vi "Power vs. MW contrast scan.vi"() -> ()   [LabVIEW 2011]
uses:
  Colton LabView code/Instruments/Laser power controller/BEOC LPC/BEOC LPC.lvlib
panel:
  out "XY Graph":cluster{"Y":dbl[], "Y":dbl[]}[](graph)
  in  "Time(s)":dbl
  in  "Power Step":dbl
  in  "Power Max":dbl
  in  "Power Min":dbl
  in  "rate":dbl=100.0 format="%0.2f"
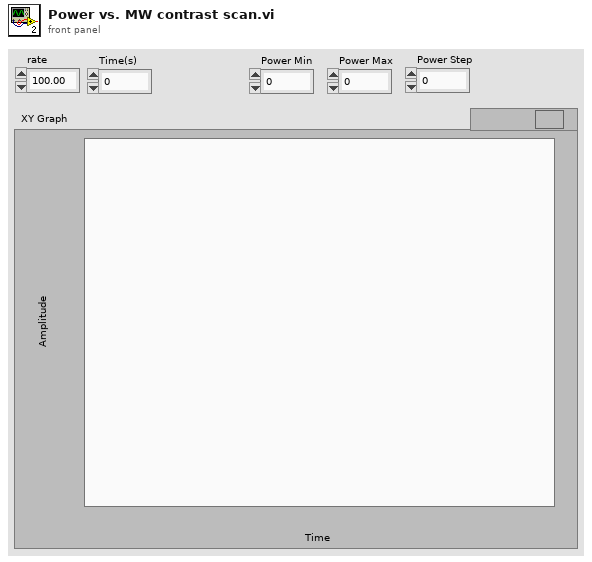
[diagram p1: front panel]
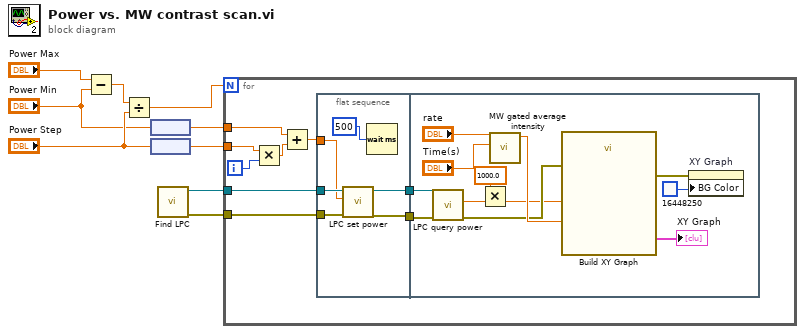
[diagram p0: block diagram]
diagram:
  n1 = Subtract(x="Power Max", y="Power Min") -> (x-y=w8:dbl)
  n2 = Divide(x=w8, y="Power Step") -> (x/y=w7:dbl)
  n3 = node("Power Min") -> (w1:dbl[unit])
  n4 = node("Power Step") -> (w3:dbl[unit])
  n5 = call "Find LPC.vi"() -> ("error out"=w5:errorcluster, "VISA resource name out"=w6:refnum<visa-resource-name>)  [unwired: 2 in, 8 out]
  n6 = for {
    N: w7 -> [_]
    tunnel: w6 -> [w18]
    tunnel: w5 -> [w17]
    tunnel: w3 -> [w15]
    tunnel: w1 -> [w13]
    i -> [w16]
    n7 = Multiply(x=w15, y=w16) -> (x*y=w14:dbl[unit])
    n8 = Add(x=w13, y=w14) -> (x+y=w12:dbl[unit])
    n9 = flat-sequence {
      tunnel: w18 -> [w24]
      tunnel: w17 -> [w23]
      tunnel: w12 -> [w22]
      tunnel: [w21] -> w11
      tunnel: [w20] -> w10
      tunnel: w11 -> [w34]
      tunnel: w10 -> [w33]
      frame #0 {
        n10 = call "LPC set power.vi"("error in (no error)"=w23, "power"=w22, "VISA resource name"=w24) -> ("error out"=w20:errorcluster, "VISA resource name out"=w21:refnum<visa-resource-name>)  [unwired: 7 in]
        n11 = Wait (ms)(milliseconds to wait=u32 500) -> ()  [unwired: 1 out]
      }
      frame #1 {
        n12 = call "LPC query power.vi"("error in (no error)"=w33, "VISA resource name"=w34) -> ("error out"=w28:errorcluster, "power"=w32:dbl[unit])  [unwired: 7 in, 1 out]
        n13 = Multiply(x=dbl[unit] 1000.0, y=w32) -> (x*y=w26:dbl[unit])
        n14 = call "MW gated average intensity.vi"("Time"="Time(s)", "rate"="rate") -> ("Contrast (%)"=w31:dbl)  [unwired: 9 in]
        n15 = call "Build XY Graph"("error in (no error)"=w28, "Y Input"=w31, "X Input"=w26) -> ("error out"=w29:errorcluster, "XY Graph"=→"XY Graph":cluster{"Y":dbl[], "Y":dbl[]}[])  [unwired: 2 in, 5 out]
        n16 = property on="XY Graph" class="XYGraph (strict)"(error in=w29, "BG Color"=u32 16448250) -> ()  [unwired: 1 in, 2 out]
      }
    }
  }
